vi "WriteTree.vi"(8 "error in":errorcluster, 11 "cRIO repo in":refnum<class "cRIORepo.lvclass">) -> (0 "error out":errorcluster, 2 "root":T1, 3 "repository out":refnum<class "NISE_CEF_Repository.lvclass">)   [LabVIEW 2015, in "cRIORepo.lvclass"]
uses:
  cRIORepo.lvclass
  <vilib>/NI/Configuration Framework/Repository/NISE_CEF_Repository.lvclass
  <vilib>/NI/Configuration Framework/Node/NodeRef.ctl
  <vilib>/NI/Configuration Framework/Node/NISE_CEF_Node.lvclass
  cRIO/cRIO.lvclass
  <vilib>/NI/Configuration Framework/hierarchy repo/NISE_CEF_HierarchyRepo.lvclass
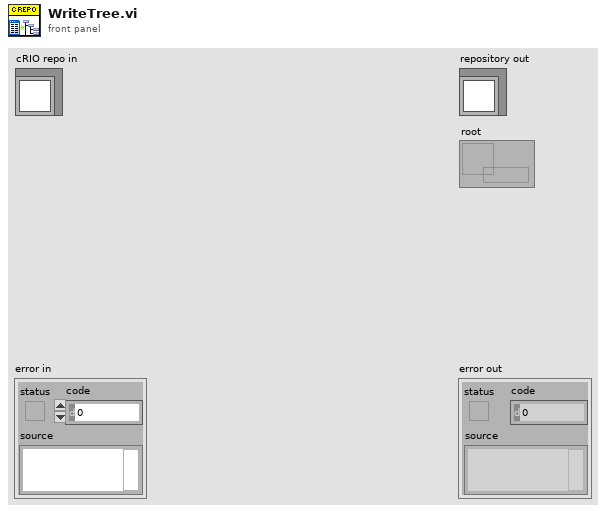
[diagram p1: front panel]
types:
  T1 = typedef "NISE_CEF_Node.lvclass/NodeRef.ctl" = refnum<data-value>
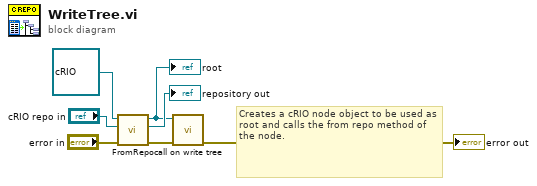
[diagram p0: block diagram]
diagram:
  # "Creates a cRIO node object to be used as root and calls the from repo method of the node."
  n1 = call-dynamic "FromRepo.vi"("error in"="error in", "repository in"="cRIO repo in", "cRIO in"=refnum<class "cRIO.lvclass"> refnum ("cRIO.lvclass")) -> ("error out"=w3:errorcluster, "repository out"=→"repository out":refnum<class "NISE_CEF_Repository.lvclass">, "node"=w2:T1)  [unwired: 6 in]
  "root" <- w2
  n2 = call <vilib>:"call on write tree.vi"("error in"=w3, "root"=w2) -> ("error out"=→"error out":errorcluster)  [unwired: 9 in]
